vi "Chain3_bak.vi"(7 "Name (\"\" to Use UUID)":string="CSM-Module") -> ()   [LabVIEW 2017, in "CSM-Testcase.lvlib"]
doc: "Creates a template for a CSM module without a user interface.\n\n> [!NOTE] CSM Name Rules\n> - The CSM module name must be unique to avoid entering the \"Critical Error\" state.\n> - If the input is \"\", a UUID will be used as the module name. This module will operate in independent mode and will not be listed in the module list.\n> - If the input ends with '#', the module will run in work mode. Modules with the same name will share the same message queue. External messages will be handled by the idle module.\n\n> [!NOTE] CSM Initialization State\n> - The default value is \"Macro: Initialize\", consistent with the JKISM state machine.\n> - This state is typically not modified and is provided to facilitate external programmatic changes to the initialization state.\n\n\n-- <b>Controls</b> --\n- <b>Name (\"\" to Use UUID)</b>: CSM Module Name\n- <b>Init State(\"Macro: Initialize\")</b>: Initialization State, default is \"Macro: Initialize\""
uses:
  CSM-Testcase.lvlib
  250f9197-eaab-42aa-85f4-d19595f3ef40.vi
  b1f9a1d7-2f6f-40c5-bed8-42b286b8eb3f.vi
  e695532a-dccc-48b0-b567-f6fcd461bdfb.vi
  src/user.lib/_NEVSTOP/Communicable State Machine(CSM)/AdvanceAPI/CSM - Revert Arguments-Safe String.vi
  src/user.lib/_NEVSTOP/Communicable State Machine(CSM)/AdvanceAPI/CSM - Make String Arguments Safe.vi
  src/user.lib/_NEVSTOP/Communicable State Machine(CSM)/AdvanceAPI/CSM - Break Down Multiple States String.vi
  src/user.lib/_NEVSTOP/Communicable State Machine(CSM)/AdvanceAPI/CSM - Keywords.vi
  src/user.lib/_NEVSTOP/Communicable State Machine(CSM)/_Shared/Trim Single-line Text.vi
  Global-TestcaseCSM.vi
  src/user.lib/_NEVSTOP/Communicable State Machine(CSM)/_Polymophic/Build No-Reply Asynchronous Message with Arguments.vi
  src/user.lib/_NEVSTOP/Communicable State Machine(CSM)/_Polymophic/Build Asynchronous Message with Arguments.vi
  src/user.lib/_NEVSTOP/Communicable State Machine(CSM)/_Polymophic/Build Register Status Message.vi
  src/user.lib/_NEVSTOP/Communicable State Machine(CSM)/Communicable State Machine.lvlib
panel:
  out "Error Occurred":errorcluster
  out "State History":string
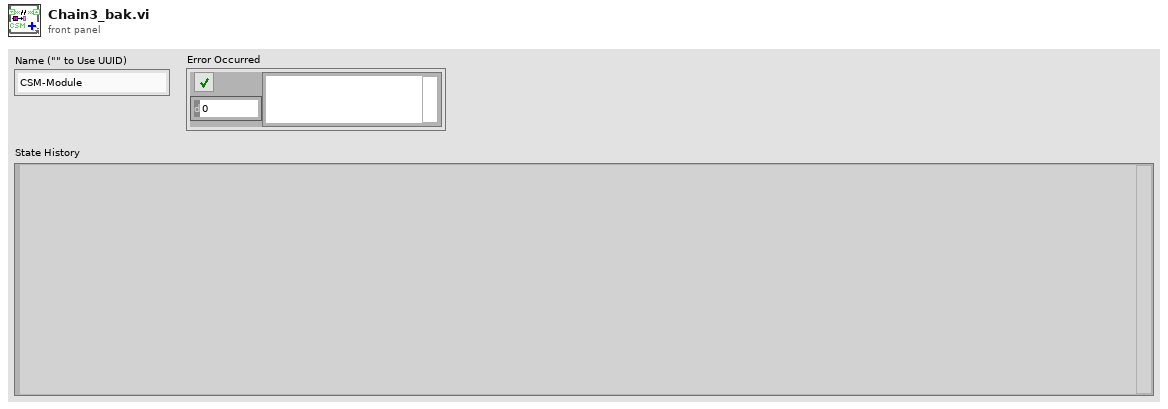
[diagram p1: front panel]
types:
  T1 = cluster{"Arguments":string, "Response":string, "error":errorcluster}
  T2 = enum32{"Invalid", "Standard", "Closed", "Hidden", "Minimized", "Maximized"}
  T3 = enum32{"invalid app kind", "Development System", "Run Time System", "Student Edition", "Embedded LabVIEW", "Evaluation", "Custom"}
  T4 = typedef "Communicable State Machine.lvlib/_CSM_Response Source Message.ctl" = cluster{"‘State":string, "’Arguments":string, "’Error":errorcluster}
  T5 = cluster{"Current VI Reference":refnum<vi>, "Close Panel on Exit?":bool}
  T6 = cluster{"Core":cluster{"Current VI Reference":refnum<vi>, "Close Panel on Exit?":bool}, "Your Boolean data":bool, "Your string data":string}
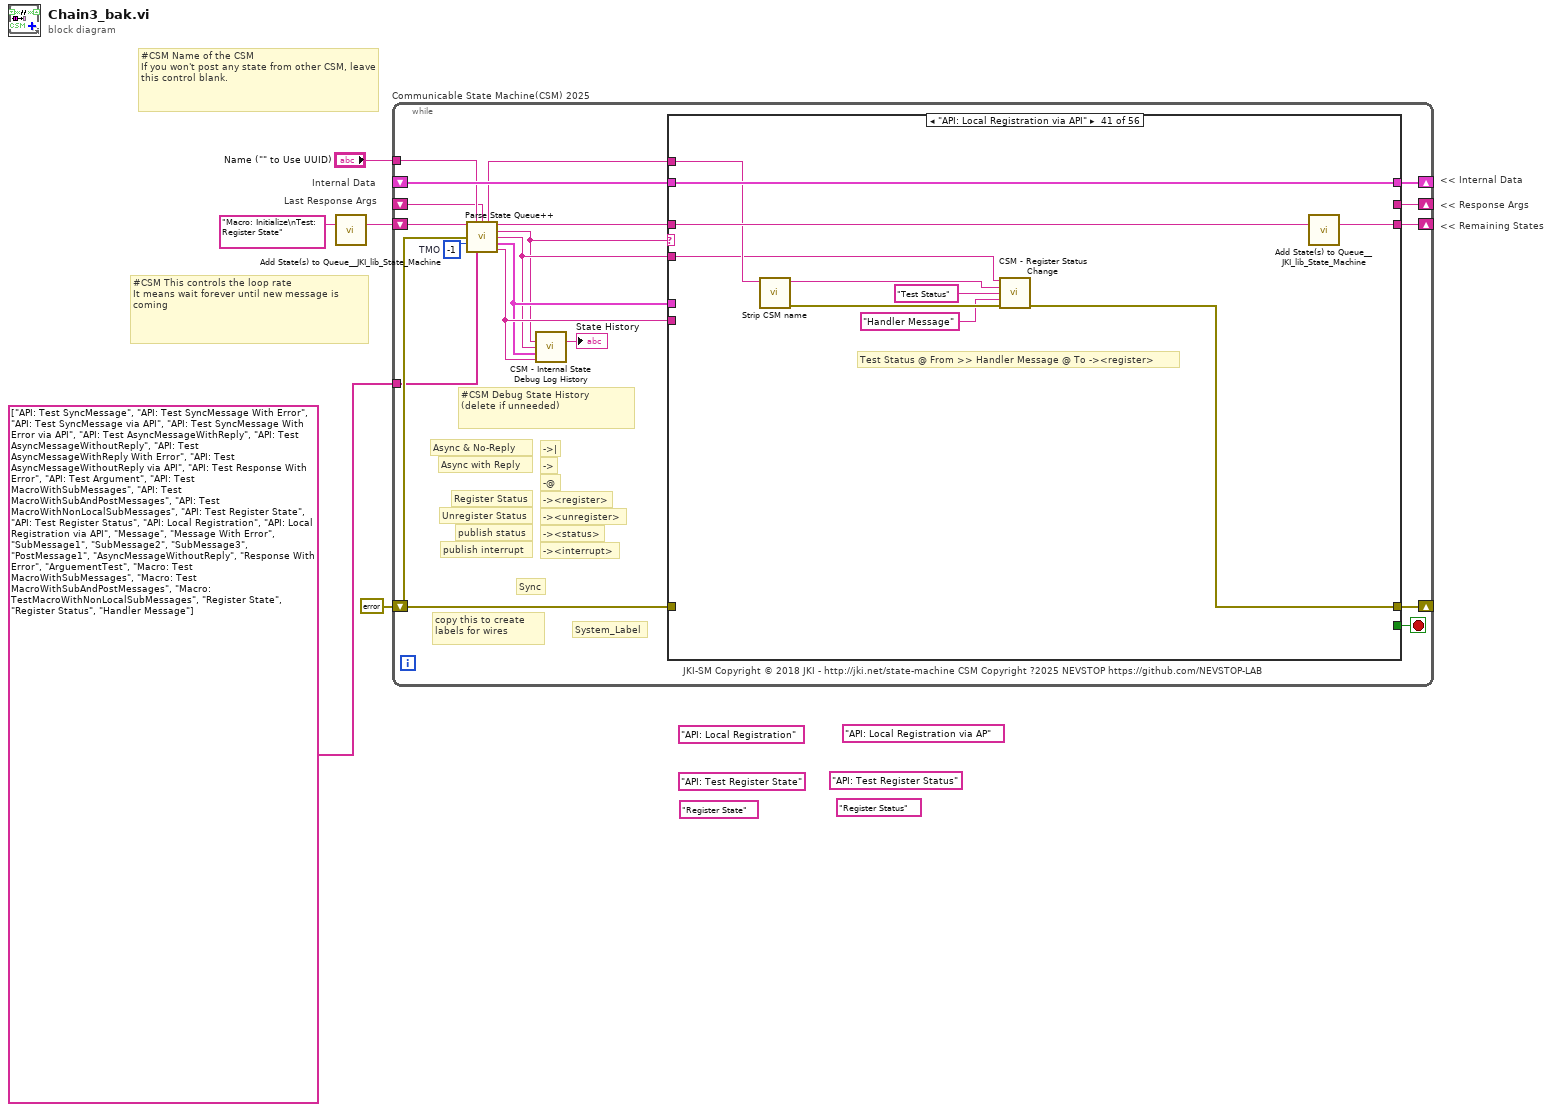
[diagram p0: block diagram]
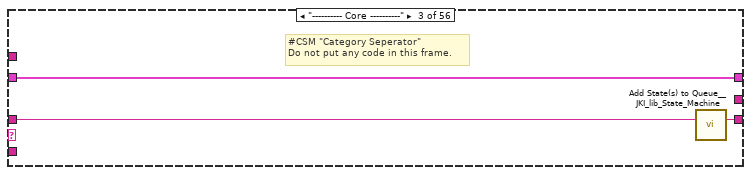
[diagram p4: hidden frame]
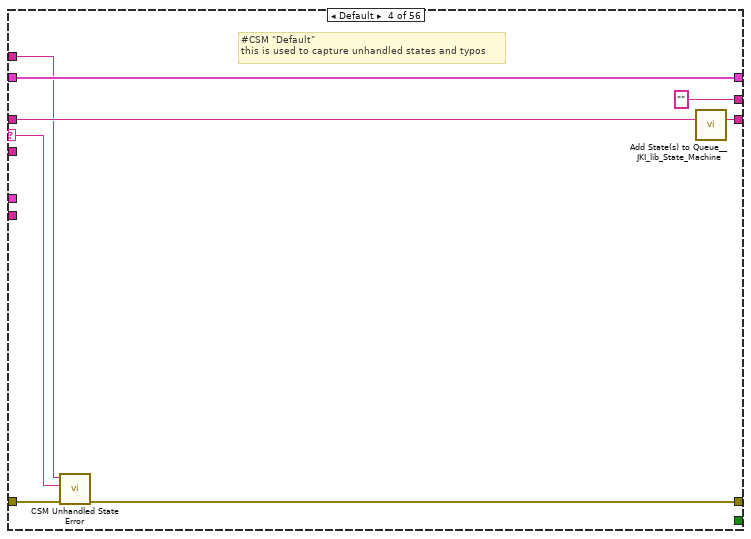
[diagram p5: hidden frame]
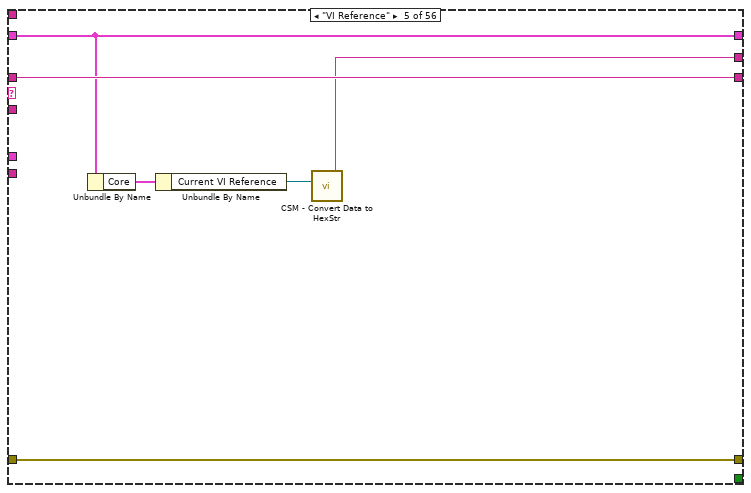
[diagram p6: hidden frame]
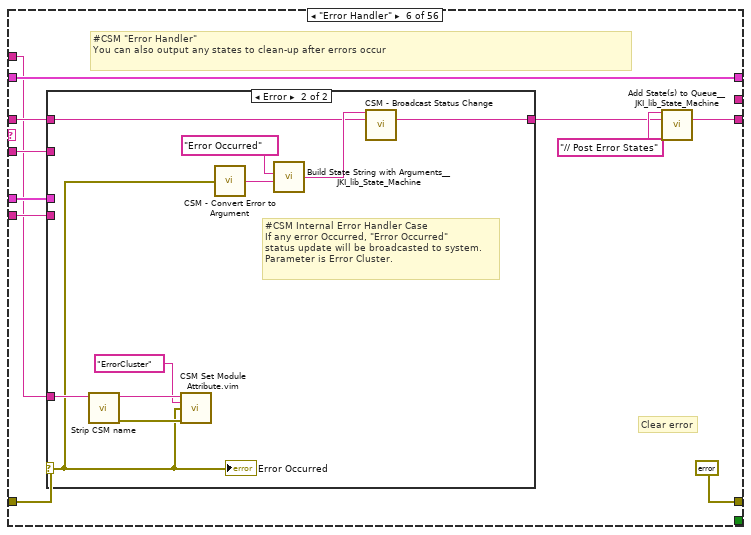
[diagram p7: hidden frame]
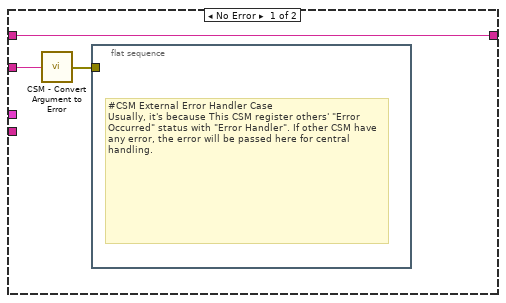
[diagram p8: hidden frame]
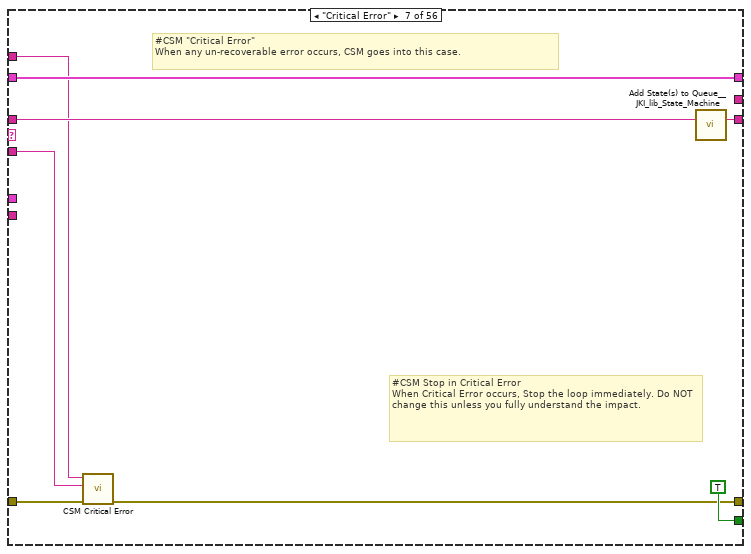
[diagram p9: hidden frame]
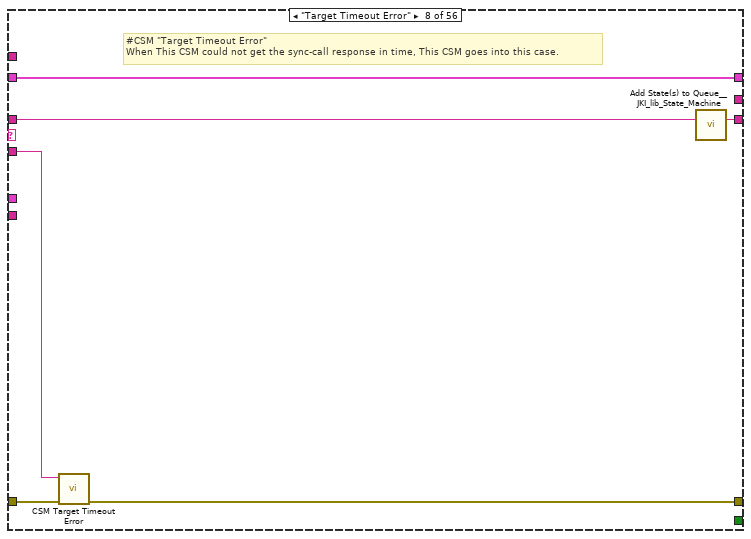
[diagram p10: hidden frame]
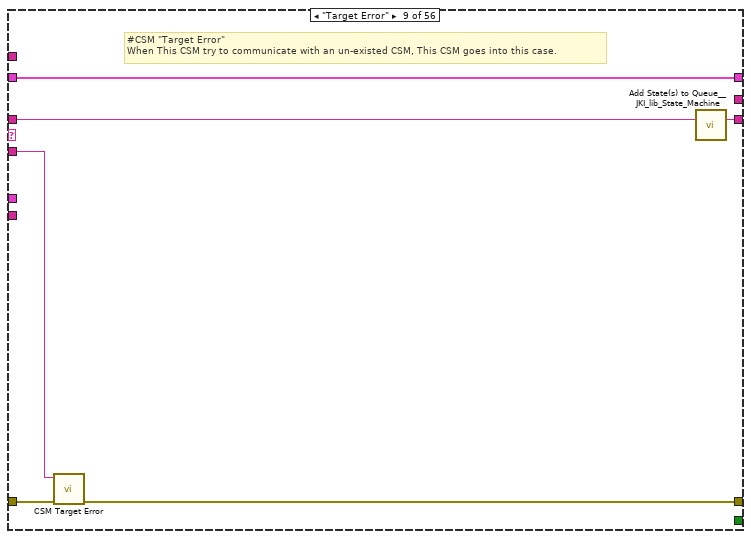
[diagram p11: hidden frame]
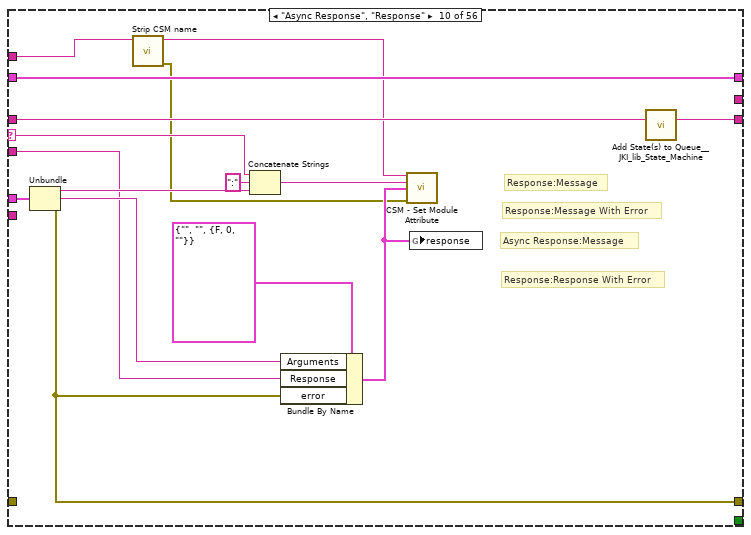
[diagram p12: hidden frame]
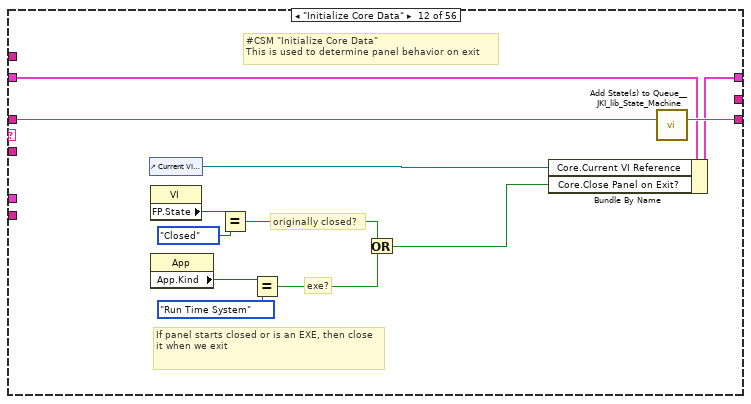
[diagram p14: hidden frame]
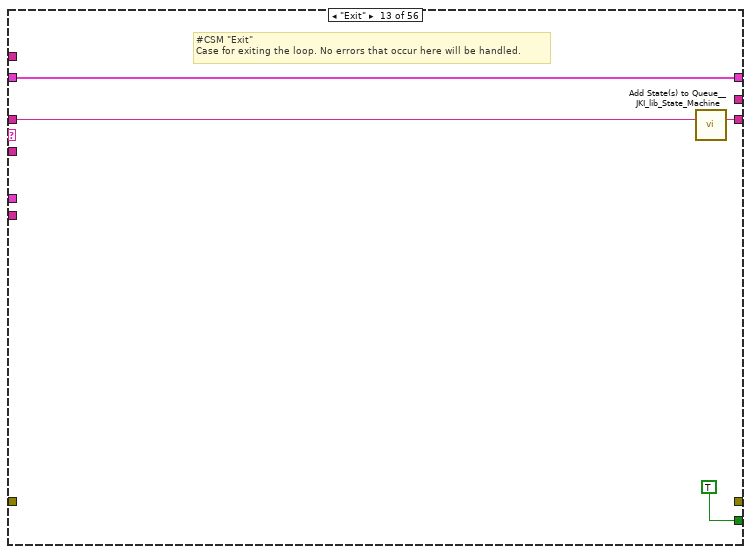
[diagram p15: hidden frame]
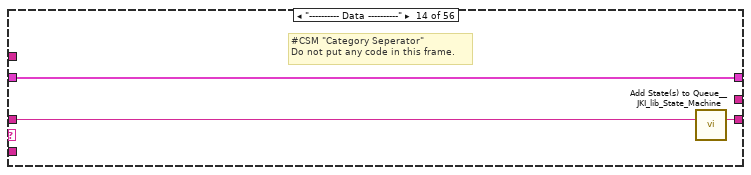
[diagram p16: hidden frame]
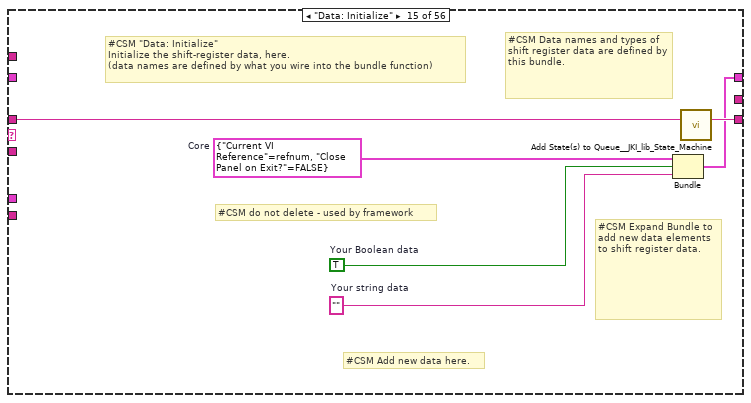
[diagram p17: hidden frame]
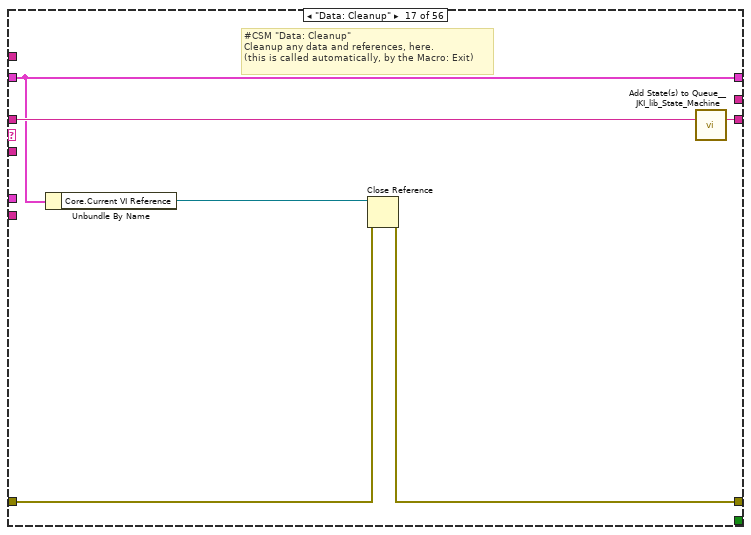
[diagram p19: hidden frame]
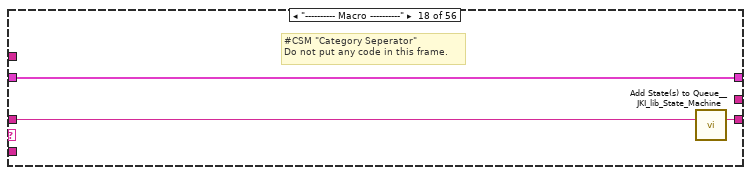
[diagram p20: hidden frame]
diagram:
  (unwired) "API: Local Registration via AP"
  (unwired) "API: Local Registration"
  (unwired) "API: Test Register Status"
  (unwired) "API: Test Register State"
  (unwired) "Register State"
  (unwired) "Register Status"
  # "Last Response Args"
  # "Internal Data"
  # "#CSM Name of the CSM\nIf you won't post any state from other CSM, leave this control blank."
  # "#CSM This controls the loop rate\nIt means wait forever until new message is coming"
  # "<< Internal Data"
  # "<< Response Args"
  # "<< Remaining States"
  n1 = call <vilib>:"Add State(s) to Queue__JKI_lib_State_Machine.vi"("State(s) in (\"\")"="Macro: Initialize\nTest: Register State" ("Init State(\"Macro: Initialize\")")) -> ("States Out"=w5:string)  [unwired: 14 in]
  n2 = while "Communicable State Machine(CSM) 2025" {
    shift-right: [w19] -> _
    shift-left: _ -> [w18]
    shift-right: [w22] -> _
    shift-left: errorcluster {"status"=FALSE, "code"=0, "source"=""} ("error out") -> [w8]
    shift-right: [w21] -> _
    shift-left: w5 -> [w23]
    tunnel: "Name (\"\" to Use UUID)" -> [w15]
    shift-right: [w16] -> _
    shift-left: _ -> [w10]
    tunnel: string[] ["API: Test SyncMessage", "API: Test SyncMessage With Error", "API: Test SyncMessage via API", "API: Test SyncMessage With Error via API", "API: Test AsyncMessageWithReply", "API: Test AsyncMessageWithoutReply", "API: Test AsyncMessageWithReply With Error", "API: Test AsyncMessageWithoutReply via API", "API: Test Response With Error", "API: Test Argument", "API: Test MacroWithSubMessages", "API: Test MacroWithSubAndPostMessages", "API: Test MacroWithNonLocalSubMessages", "API: Test Register State", "API: Test Register Status", "API: Local Registration", "API: Local Registration via API", "Message", "Message With Error", "SubMessage1", "SubMessage2", "SubMessage3", "PostMessage1", "AsyncMessageWithoutReply", "Response With Error", "ArguementTest", "Macro: Test MacroWithSubMessages", "Macro: Test MacroWithSubAndPostMessages", "Macro: TestMacroWithNonLocalSubMessages", "Register State", "Register Status", "Handler Message"] ("Allowed Messages (Empty for All)") -> [w6]
    stop <- w20 stop-if-true
    w17 = -1  # TMO
    # "#CSM Debug State History\n(delete if unneeded)"
    # "-><interrupt>"
    # "-><status>"
    # "-><unregister>"
    # "-><register>"
    # "-@"
    # "->"
    # "->|"
    # "publish interrupt"
    # "publish status"
    # "Unregister Status"
    # "Register Status"
    # "Sync"
    # "Async with Reply"
    # "Async & No-Reply"
    # "JKI-SM Copyright © 2018 JKI - http://jki.net/state-machine CSM Copyright ?2025 NEVSTOP https://github.com/NEVSTOP-LAB"
    # "copy this to create labels for wires"
    # "System_Label"
    n3 = call "Parse State Queue++.vi"("State Queue"=w23, "Name (\"\" to Use UUID)"=w15, "Response Arguments"=w10, "Previous Error"=w8, "Dequeue (1 ms)"=w17, "Allowed Messages (Empty for All)"=w6) -> ("Name Used"=w9:string, "Remaining States"=w24:string, "Current State"=w11:string, "Arguments"=w12:string, ">> Response Source Message >>"=w13:T4, ">> Source CSM >>"=w14:string)  [unwired: 4 in]
    n4 = call "CSM - Internal State Debug Log History.vi"("State"=w11, "Arguments (\"\")"=w12, ">> Response Source Message >>"=w13, "Source (\"\")"=w14) -> ("Debug Log"=→"State History":string)  [unwired: 11 in]
    n5 = case shown="\"API: Local Registration via API\"" w11 {
      selector: w11 -> [_ _ _ w35 _ _ _ _ _ w101 _ _ _ _ _ _ _ _ _ _ _ _ _ _ _ _ _ _ _ _ _ _ _ _ _ _ _ _ _ _ _ _ _ _ _ _ _ _ _ w487 _ _ _ w512 w525 w531]
      tunnel: w24 -> [w25 w28 w31 w39 w44 w50 w77 w83 w89 w105 w107 w119 w123 w126 w132 w134 w140 w143 w147 w153 w167 w187 w216 w220 w224 w236 w264 w296 w312 w324 w336 w350 w373 w384 w397 w404 w411 w418 w425 w437 w447 w451 w456 w459 w465 w470 w473 w477 w481 w491 w495 w503 w509 w517 w527 w537]
      tunnel: w12 -> [_ _ _ _ _ w49 w73 w80 w86 w95 _ _ _ _ _ _ _ _ _ _ w154 w174 w199 _ w227 w239 w267 w299 w315 w327 w339 w353 w369 w387 w394 w401 w408 w415 w422 w429 w438 w449 _ _ w461 w466 w472 w476 w480 w486 w494 w501 w507 w514 w526 w530]
      tunnel: w18 -> [w26 w27 w29 w37 w43 w55 w75 w81 w87 w103 w106 w113 w121 w124 _ w133 w135 w141 w145 w151 w169 w189 w218 w219 w228 w240 w268 w300 w316 w328 w340 w354 w376 w388 w399 w406 w413 w420 w427 w435 w445 w450 w454 w457 w463 w471 w474 w478 w482 w492 w496 w502 w508 w518 w528 w538]
      tunnel: [_ _ _ w32 w45 errorcluster {"status"=FALSE, "code"=0, "source"=""} ("error out") w70 w78 w84 w94 _ _ _ _ _ _ w136 _ _ _ _ _ _ _ w221 w233 w261 w293 w309 w321 w333 w346 w370 w381 w398 w405 w412 w419 w426 w431 w442 _ _ _ _ _ w475 w479 w483 w485 w497 w498 w504 w511 w521 w533] -> w22
      tunnel: w8 -> [_ _ _ w33 w45 w53 w71 w79 w85 _ _ _ _ _ _ _ w137 _ _ _ _ _ _ _ _ _ _ _ _ _ _ _ _ _ w398 w405 w412 w419 w426 _ _ _ _ _ _ _ w475 w479 w483 w493 w497 w499 w505 w519 w529 w539]
      tunnel: [w25 w28 w30 w38 w44 w51 w76 w82 w88 w104 w107 w118 w122 w125 w131 w134 w139 w142 w146 w152 w168 w188 w217 w220 w225 w237 w265 w297 w313 w325 w337 w351 w374 w385 w396 w403 w410 w417 w424 w436 w446 w451 w455 w458 w464 w467 w473 w477 w481 w491 w495 w503 w509 w517 w527 w537] -> w21
      tunnel: [_ _ _ _ _ _ TRUE _ _ _ _ _ TRUE _ _ _ _ _ _ _ _ _ _ _ _ _ _ _ _ _ _ _ _ _ _ _ _ _ _ _ _ _ _ _ _ _ _ _ _ _ _ _ _ _ _ _] -> w20
      tunnel: [w26 w27 w29 w37 w43 w55 w75 w81 w87 w103 w106 w117 w121 w124 w130 w133 w135 w141 w145 w151 w169 w189 w218 w219 w228 w240 w268 w300 w316 w328 w340 w354 w376 w388 w399 w406 w413 w420 w427 w435 w445 w450 w454 w457 w463 w471 w474 w478 w482 w492 w496 w502 w508 w518 w528 w538] -> w19
      tunnel: w14 -> [_ _ _ _ _ w48 _ _ _ _ _ _ _ _ _ _ _ _ _ _ _ _ _ _ _ _ _ _ _ _ _ _ _ _ _ _ _ _ _ _ _ _ _ _ _ _ _ _ _ _ _ _ _ _ _ _]
      tunnel: w13 -> [_ _ _ _ _ w47 _ _ _ w102 _ _ _ _ _ _ _ _ _ _ _ _ _ _ _ _ _ _ _ _ _ _ _ _ _ _ _ _ _ _ _ _ _ _ _ _ _ _ _ _ _ _ _ _ _ _]
      tunnel: [_ _ _ "" w40 _ _ _ _ _ _ _ _ _ _ _ _ _ _ _ _ _ _ _ _ _ _ _ _ _ _ _ _ _ _ _ _ _ _ _ _ w448 _ _ _ _ w472 w476 w480 w486 w494 w501 w507 _ w526 w530] -> w16
      tunnel: w9 -> [_ _ _ w34 _ w46 w72 _ _ w92 _ _ _ _ _ _ _ _ _ _ _ _ _ _ _ _ w252 w284 _ _ _ w347 _ _ _ _ _ _ _ w433 w444 _ _ _ _ _ _ _ _ w490 _ _ _ w516 w524 w536]
      frame "", "Idle" {
        # "#CSM \"Idle/Event Handler\"\nexecutes when the state queue is empty"
      }
      frame "CSM Documentation" {
        # "#CSM State Syntax\n\n// Comment line, all text to the right of “//” will be ignored\n// Local Message Example\nDoSth: DoA >> Arguments\n\n// Sync Call Example\nAPI: xxxx >> Arguments -@ TargetModule\n\n// Async Call Example\nAPI: xxxx >> Arguments -> TargetModule\n\n// Async Call without Reply Example\nAPI: xxxx >> Arguments ->| TargetModule\n\n// Broadcast normal status:\nStatus >> StatusArguments  -><status>\n\n// Broadcast Interrupt status:\nInterrupt >> StatusArguments  -><interrupt>\n\n// Register Source Module's status to Handler Module\nStatus@Source Module >> Handler Module@Handler Module -><register>\n\n// Unegister Source Module's status\nStatus@Source Module >> Handler Module -><unregister>"
        # "#CSM README FIRST\n\nCommunicable State Machine(CSM) is a LabVIEW application framework that builds upon JKI State Machine(JKISM). It follows the pattern of JKISM and extends the keywords to describe message communication between modules, including concepts such as Sync-Message, Async-Message, Subscription/Unsubscription of status - essential elements for creating reusable code modules. For more information, please visit the CSM wiki: https://nevstop-lab.github.io/CSM-Wiki/\n\nFor instructions on JKI State Machine, visit: \n    http://jki.net/state-machine/\nFor information about CSM, visit: \n    https://github.com/NEVSTOP-LAB"
        # "#CSM \"Documentation\"\nCase for holding CSM Documenation"
      }
      frame "---------- Core ----------" {
        # "#CSM \"Category Seperator\"\nDo not put any code in this frame."
        n6 = call <vilib>:"Add State(s) to Queue__JKI_lib_State_Machine.vi"("State(s) in (\"\")"=w31) -> ("States Out"=w30:string)  [unwired: 14 in]
      }
      frame Default {
        # "#CSM \"Default\"\nthis is used to capture unhandled states and typos"
        n7 = call "CSM Unhandled State Error.vi"("error in (no error)"=w33, "Current State"=w35, "CSM Name"=w34) -> ("error out"=w32:errorcluster)  [unwired: 8 in]
        n8 = call <vilib>:"Add State(s) to Queue__JKI_lib_State_Machine.vi"("State(s) in (\"\")"=w39) -> ("States Out"=w38:string)  [unwired: 14 in]
      }
      frame "VI Reference" {
        n9 = Unbundle By Name(w43) -> ("Core"=w42:T5)
        n10 = Unbundle By Name(w42) -> ("Current VI Reference"=w41:refnum<vi>)
        n11 = call "CSM - Convert Data to HexStr.vi"("Variant"=w41) -> ("HEX String (0-9,A-F)"=w40:string)  [unwired: 8 in]
      }
      frame "Error Handler" {
        # "#CSM \"Error Handler\"\nYou can also output any states to clean-up after errors occur"
        # "Clear error"
        n12 = case shown="Error" w53 {
          selector: w53 -> [_ w61]
          tunnel: [w59 w66] -> w52
          tunnel: w50 -> [w59 w65]
          tunnel: w49 -> [w58 _]
          tunnel: w48 -> [_ _]
          tunnel: w47 -> [_ _]
          tunnel: w46 -> [_ w64]
          frame No Error {
            n13 = call "CSM - Convert Argument to Error.vi"("Argument"=w58) -> ("Error"=w57:errorcluster)  [unwired: 4 in]
            n14 = flat-sequence {
              tunnel: w57 -> [_]
              frame #0 {
                # "#CSM External Error Handler Case\nUsually, it's because This CSM register others' \"Error Occurred\" status with \"Error Handler\". If other CSM have any error, the error will be passed here for central handling."
              }
            }
          }
          frame Error {
            # "#CSM Internal Error Handler Case \nIf any error Occurred, \"Error Occurred\" \nstatus update will be broadcasted to system.\nParameter is Error Cluster."
            n15 = call "Strip CSM name.vi"("CSM name"=w64) -> ("error out"=w63:errorcluster, "CSM name core"=w62:string)  [unwired: 7 in, 2 out]
            n16 = call "CSM Set Module Attribute.vim"("CSM Name"=w62, "Attribute"="ErrorCluster", "Value"=w61, "Error In"=w63) -> ()  [unwired: 8 in, 4 out]
            n17 = call "CSM - Convert Error to Argument.vi"("Error"=w61) -> ("Argument"=w68:string)  [unwired: 4 in]
            n18 = call <vilib>:"Build State String with Arguments__JKI_lib_State_Machine.vi"("Arguments (\"\")"=w68, "State"="Error Occurred" ("Status with Arguments")) -> ("State with Arguments"=w67:string)  [unwired: 4 in]
            n19 = call "CSM - Broadcast Status Change.vi"("Status With Arguments"=w67, "State Queue"=w65) -> ("Remaining States"=w66:string)  [unwired: 13 in]
            "Error Occurred" <- w61
          }
        }
        n20 = call <vilib>:"Add State(s) to Queue__JKI_lib_State_Machine.vi"("State(s) in Front (\"\")"="// Post Error States", "State(s) in (\"\")"=w52) -> ("States Out"=w51:string)  [unwired: 13 in]
      }
      frame "Critical Error" {
        # "#CSM \"Critical Error\"\nWhen any un-recoverable error occurs, CSM goes into this case."
        # "#CSM Stop in Critical Error\nWhen Critical Error occurs, Stop the loop immediately. Do NOT change this unless you fully understand the impact."
        n21 = call "CSM Critical Error.vi"("error in (no error)"=w71, "Arugments (As Reason)"=w73, "CSM Name"=w72) -> ("error out"=w70:errorcluster)  [unwired: 8 in]
        n22 = call <vilib>:"Add State(s) to Queue__JKI_lib_State_Machine.vi"("State(s) in (\"\")"=w77) -> ("States Out"=w76:string)  [unwired: 14 in]
      }
      frame "Target Timeout Error" {
        # "#CSM \"Target Timeout Error\"\nWhen This CSM could not get the sync-call response in time, This CSM goes into this case."
        n23 = call "CSM Target Timeout Error.vi"("error in (no error)"=w79, "Arguments (As CSM Name)"=w80) -> ("error out"=w78:errorcluster)  [unwired: 9 in]
        n24 = call <vilib>:"Add State(s) to Queue__JKI_lib_State_Machine.vi"("State(s) in (\"\")"=w83) -> ("States Out"=w82:string)  [unwired: 14 in]
      }
      frame "Target Error" {
        # "#CSM \"Target Error\"\nWhen This CSM try to communicate with an un-existed CSM, This CSM goes into this case."
        n25 = call "CSM Target Error.vi"("error in (no error)"=w85, "Arguments (As CSM Name)"=w86) -> ("error out"=w84:errorcluster)  [unwired: 9 in]
        n26 = call <vilib>:"Add State(s) to Queue__JKI_lib_State_Machine.vi"("State(s) in (\"\")"=w89) -> ("States Out"=w88:string)  [unwired: 14 in]
      }
      frame "Async Response", "Response" {
        # "Response:Response With Error"
        # "Response:Message With Error"
        # "Async Response:Message"
        # "Response:Message"
        n27 = Unbundle(w102) -> ("‘State"=w100:string, "’Arguments"=w96:string, "’Error"=w94:errorcluster)
        n28 = call "Strip CSM name.vi"("CSM name"=w92) -> ("error out"=w90:errorcluster, "CSM name core"=w91:string)  [unwired: 7 in, 2 out]
        n29 = Concatenate Strings(w101, ":" ("string"), w100) -> (w98:string)
        n30 = Bundle By Name(cluster=T1 {"Arguments"="", "Response"="", "error"={"status"=FALSE, "code"=0, "source"=""}}, "Arguments"=w96, "Response"=w95, "error"=w94) -> (w93:T1)
        n31 = call "CSM - Set Module Attribute.vi"("CSM Name"=w91, "Attribute"=w98, "Value"=w93, "Error In"=w90) -> ()  [unwired: 8 in, 4 out]
        n32 = global write "Global-TestcaseCSM.vi" "response"(w93) -> ()
        n33 = call <vilib>:"Add State(s) to Queue__JKI_lib_State_Machine.vi"("State(s) in (\"\")"=w105) -> ("States Out"=w104:string)  [unwired: 14 in]
      }
      frame "Async Message Posted" {
        # "#CSM \"Async Message Posted\"\nAfter Async Message is posted (-> or ->| ), CSM goes to this state for post-action.\nYou can use Argument - State to tell which Async Message is called."
      }
      frame "Initialize Core Data" {
        # "#CSM \"Initialize Core Data\"\nThis is used to determine panel behavior on exit"
        # "originally closed?"
        # "exe?"
        # "If panel starts closed or is an EXE, then close it when we exit"
        n34 = control-ref of="Current VI Reference"() -> (w111:refnum<vi>)
        n35 = property class="VI"() -> ("FP.State"=w110:T2)  [unwired: 2 in, 2 out]
        n36 = property class="App"() -> ("App.Kind"=w116:T3)  [unwired: 2 in, 2 out]
        n37 = Equal?(x=w110, y=T2."Closed" ("Front Panel Window:State")) -> (x = y?=w108:bool)
        n38 = Equal?(x=w116, y=T3."Run Time System" ("Application:Kind")) -> (x = y?=w114:bool)
        n39 = Or(x=w108, y=w114) -> (x .or. y?=w112:bool)
        n40 = Bundle By Name(cluster=w113, "Core.Current VI Reference"=w111, "Core.Close Panel on Exit?"=w112) -> (w117:T6)
        n41 = call <vilib>:"Add State(s) to Queue__JKI_lib_State_Machine.vi"("State(s) in (\"\")"=w119) -> ("States Out"=w118:string)  [unwired: 14 in]
      }
      frame "Exit" {
        # "#CSM \"Exit\"\nCase for exiting the loop. No errors that occur here will be handled."
        n42 = call <vilib>:"Add State(s) to Queue__JKI_lib_State_Machine.vi"("State(s) in (\"\")"=w123) -> ("States Out"=w122:string)  [unwired: 14 in]
      }
      frame "---------- Data ----------" {
        # "#CSM \"Category Seperator\"\nDo not put any code in this frame."
        n43 = call <vilib>:"Add State(s) to Queue__JKI_lib_State_Machine.vi"("State(s) in (\"\")"=w126) -> ("States Out"=w125:string)  [unwired: 14 in]
      }
      frame "Data: Initialize" {
        w127 = T5 {"Current VI Reference"=refnum, "Close Panel on Exit?"=FALSE}  # Core
        w129 = TRUE  # Your Boolean data
        w128 = ""  # Your string data
        # "#CSM \"Data: Initialize\"\nInitialize the shift-register data, here.\n(data names are defined by what you wire into the bundle function)"
        # "#CSM do not delete - used by framework"
        # "#CSM Expand Bundle to add new data elements to shift register data."
        # "#CSM Add new data here."
        # "#CSM Data names and types of shift register data are defined by this bundle."
        n44 = Bundle("Core"=w127, "Your Boolean data"=w129, "Your string data"=w128) -> (w130:T6)  [unwired: 1 in]
        n45 = call <vilib>:"Add State(s) to Queue__JKI_lib_State_Machine.vi"("State(s) in (\"\")"=w132) -> ("States Out"=w131:string)  [unwired: 14 in]
      }
      frame "Data: Update Indicators" {
      }
      frame "Data: Cleanup" {
        # "#CSM \"Data: Cleanup\"\nCleanup any data and references, here.\n(this is called automatically, by the Macro: Exit)"
        n46 = Unbundle By Name(w135) -> ("Core.Current VI Reference"=w138:refnum<vi>)
        n47 = Close Reference(reference=w138, error in (no error)=w137) -> (error out=w136:errorcluster)
        n48 = call <vilib>:"Add State(s) to Queue__JKI_lib_State_Machine.vi"("State(s) in (\"\")"=w140) -> ("States Out"=w139:string)  [unwired: 14 in]
      }
      frame "---------- Macro ----------" {
        # "#CSM \"Category Seperator\"\nDo not put any code in this frame."
        n49 = call <vilib>:"Add State(s) to Queue__JKI_lib_State_Machine.vi"("State(s) in (\"\")"=w143) -> ("States Out"=w142:string)  [unwired: 14 in]
      }
      frame "Macro: Initialize" {
        # "#CSM \"Macro: Initialize\"\nInitialization Macro (This is called once, when the VI starts)"
        n50 = call <vilib>:"Add State(s) to Queue__JKI_lib_State_Machine.vi"("State(s) in Front (\"\")"="Data: Initialize\nInitialize Core Data\nData: Update Indicators", "State(s) in (\"\")"=w147) -> ("States Out"=w146:string)  [unwired: 13 in]
      }
      frame "Macro: Exit" {
        # "#CSM \"Macro: Exit\"\nExit Macro (This is called once, when the VI exits)"
        n51 = call <vilib>:"Add State(s) to Queue__JKI_lib_State_Machine.vi"("State(s) in Front (\"\")"="//Exit Sub-Modules ", "State(s) at Back (\"\")"="Data: Cleanup\nExit") -> ("States Out"=w149:string)  [unwired: 13 in]
        n52 = call <vilib>:"Add State(s) to Queue__JKI_lib_State_Machine.vi"("State(s) in Front (\"\")"=w149, "State(s) in (\"\")"=w153) -> ("States Out"=w152:string)  [unwired: 13 in]
      }
      frame "Macro: Test MacroWithSubMessages" {
        w155 = "SubMessage2" ("State With Arguments")
        w157 = "SubMessage1" ("State With Arguments")
        n53 = call "uuid.vi"() -> ("UUID"=w156:string)  [unwired: 11 in]
        n54 = call "uuid.vi"() -> ("UUID"=w158:string)  [unwired: 11 in]
        n55 = Concatenate Strings(w157, w158) -> (w159:string)
        n56 = Concatenate Strings(w155, w156) -> (w160:string)
        n57 = call <vilib>:"Build State String with Arguments__JKI_lib_State_Machine.vi"("Arguments (\"\")"=w154, "State"="SubMessage3" ("State With Arguments")) -> ("State with Arguments"=w162:string)  [unwired: 4 in]
        n58 = call <vilib>:"Build State String with Arguments__JKI_lib_State_Machine.vi"("Arguments (\"\")"=w159, "State"=w157) -> ("State with Arguments"=w164:string)  [unwired: 4 in]
        n59 = call <vilib>:"Build State String with Arguments__JKI_lib_State_Machine.vi"("Arguments (\"\")"=w160, "State"=w155) -> ("State with Arguments"=w163:string)  [unwired: 4 in]
        n60 = Build Array(w164, w163, w162) -> (w161:string[])
        n61 = call "CSM - Compact Multiple States.vi"("Multiple States"=w161) -> ("States"=w166:string)  [unwired: 9 in]
        n62 = call <vilib>:"Add State(s) to Queue__JKI_lib_State_Machine.vi"("State(s) in Front (\"\")"=w166, "State(s) in (\"\")"=w167) -> ("States Out"=w168:string)  [unwired: 13 in]
      }
      frame "Macro: Test MacroWithSubAndPostMessages" {
        w173 = "PostMessage1" ("State With Arguments")
        w175 = "SubMessage2" ("State With Arguments")
        w177 = "SubMessage1" ("State With Arguments")
        n63 = call "uuid.vi"() -> ("UUID"=w176:string)  [unwired: 11 in]
        n64 = call "uuid.vi"() -> ("UUID"=w172:string)  [unwired: 11 in]
        n65 = call "uuid.vi"() -> ("UUID"=w178:string)  [unwired: 11 in]
        n66 = Concatenate Strings(w173, w172) -> (w171:string)
        n67 = Concatenate Strings(w177, w178) -> (w179:string)
        n68 = Concatenate Strings(w175, w176) -> (w180:string)
        n69 = call <vilib>:"Build State String with Arguments__JKI_lib_State_Machine.vi"("Arguments (\"\")"=w174, "State"="SubMessage3" ("State With Arguments")) -> ("State with Arguments"=w182:string)  [unwired: 4 in]
        n70 = call <vilib>:"Build State String with Arguments__JKI_lib_State_Machine.vi"("Arguments (\"\")"=w171, "State"=w173) -> ("State with Arguments"=w170:string)  [unwired: 4 in]
        n71 = call <vilib>:"Build State String with Arguments__JKI_lib_State_Machine.vi"("Arguments (\"\")"=w179, "State"=w177) -> ("State with Arguments"=w184:string)  [unwired: 4 in]
        n72 = call <vilib>:"Build State String with Arguments__JKI_lib_State_Machine.vi"("Arguments (\"\")"=w180, "State"=w175) -> ("State with Arguments"=w183:string)  [unwired: 4 in]
        n73 = Build Array(w184, w183, w182) -> (w181:string[])
        n74 = call "CSM - Compact Multiple States.vi"("Multiple States"=w181) -> ("States"=w186:string)  [unwired: 9 in]
        n75 = call <vilib>:"Add State(s) to Queue__JKI_lib_State_Machine.vi"("State(s) in Front (\"\")"=w186, "State(s) in (\"\")"=w187, "State(s) at Back (\"\")"=w170) -> ("States Out"=w188:string)  [unwired: 12 in]
      }
      frame "Macro: TestMacroWithNonLocalSubMessages" {
        w203 = "PostMessage1" ("State With Arguments")
        w204 = "SubMessage2" ("State With Arguments")
        w206 = "SubMessage1" ("State With Arguments")
        n76 = Match Pattern(string=w199, regular expression="+") -> (before substring=w191:string, after substring=w190:string)  [unwired: 1 in, 2 out]
        n77 = call "uuid.vi"() -> ("UUID"=w202:string)  [unwired: 11 in]
        n78 = call "uuid.vi"() -> ("UUID"=w205:string)  [unwired: 11 in]
        n79 = call "uuid.vi"() -> ("UUID"=w207:string)  [unwired: 11 in]
        n80 = Concatenate Strings(w203, w202) -> (w201:string)
        n81 = Concatenate Strings(w206, w207) -> (w208:string)
        n82 = Concatenate Strings(w204, w205) -> (w209:string)
        n83 = call <vilib>:"Build State String with Arguments__JKI_lib_State_Machine.vi"("Arguments (\"\")"=w201, "State"=w203) -> ("State with Arguments"=w200:string)  [unwired: 4 in]
        n84 = call-poly "Build Message with Arguments++.vi"("State With Arguments"="SubMessage1", "Target Module (\"\")"=w190) -> ("CSM Message String"=w195:string)  [unwired: 13 in]
        n85 = call-poly "Build Message with Arguments++.vi"("State With Arguments"="SubMessage2", "Target Module (\"\")"=w190) -> ("CSM Message String"=w194:string)  [unwired: 13 in]
        n86 = call <vilib>:"Build State String with Arguments__JKI_lib_State_Machine.vi"("Arguments (\"\")"=w191, "State"="SubMessage3" ("State With Arguments")) -> ("State with Arguments"=w211:string)  [unwired: 4 in]
        n87 = call-poly "Build Message with Arguments++.vi"("State With Arguments"="Message", "Target Module (\"\")"=w190) -> ("CSM Message String"=w196:string)  [unwired: 13 in]
        n88 = call <vilib>:"Build State String with Arguments__JKI_lib_State_Machine.vi"("Arguments (\"\")"=w208, "State"=w206) -> ("State with Arguments"=w213:string)  [unwired: 4 in]
        n89 = call <vilib>:"Build State String with Arguments__JKI_lib_State_Machine.vi"("Arguments (\"\")"=w209, "State"=w204) -> ("State with Arguments"=w212:string)  [unwired: 4 in]
        n90 = Build Array(w213, w212, w211, w196, w195, w194) -> (w210:string[])
        n91 = call "CSM - Compact Multiple States.vi"("Multiple States"=w210) -> ("States"=w215:string)  [unwired: 9 in]
        n92 = call <vilib>:"Add State(s) to Queue__JKI_lib_State_Machine.vi"("State(s) in Front (\"\")"=w215, "State(s) in (\"\")"=w216, "State(s) at Back (\"\")"=w200) -> ("States Out"=w217:string)  [unwired: 12 in]
      }
      frame "---------- API ----------" {
        # "#CSM \"Category Seperator\"\nDo not put any code in this frame."
      }
      frame "API: Test SyncMessage" {
        n93 = call "CSM - Check If Module Exists.vi"("CSM Name"=w227) -> ("error out"=w221:errorcluster, "Exist?"=w222:bool, "CSM Name (Dup)"=w226:string)  [unwired: 8 in]
        n94 = case shown="True" w222 {
          tunnel: w226 -> [_ w230]
          tunnel: [_ w229] -> w223
          frame False {
          }
          frame True {
            n95 = call "uuid.vi"() -> ("UUID"=w231:string)  [unwired: 11 in]
            n96 = call "Build Synchronous Message with Arguments.vi"("State With Arguments"="Message", "Arguments (\"\")"=w231, "Target Module (\"\")"=w230) -> ("CSM Message String"=w229:string)  [unwired: 12 in]
          }
        }
        n97 = call <vilib>:"Add State(s) to Queue__JKI_lib_State_Machine.vi"("State(s) in Front (\"\")"=w223, "State(s) in (\"\")"=w224) -> ("States Out"=w225:string)  [unwired: 13 in]
      }
      frame "API: Test SyncMessage With Error" {
        n98 = call "CSM - Check If Module Exists.vi"("CSM Name"=w239) -> ("error out"=w233:errorcluster, "Exist?"=w234:bool, "CSM Name (Dup)"=w238:string)  [unwired: 8 in]
        n99 = case shown="True" w234 {
          tunnel: w238 -> [_ w242]
          tunnel: [_ w241] -> w235
          frame False {
          }
          frame True {
            n100 = call "uuid.vi"() -> ("UUID"=w243:string)  [unwired: 11 in]
            n101 = call "Build Synchronous Message with Arguments.vi"("State With Arguments"="Message With Error", "Arguments (\"\")"=w243, "Target Module (\"\")"=w242) -> ("CSM Message String"=w241:string)  [unwired: 12 in]
          }
        }
        n102 = call <vilib>:"Add State(s) to Queue__JKI_lib_State_Machine.vi"("State(s) in Front (\"\")"=w235, "State(s) in (\"\")"=w236) -> ("States Out"=w237:string)  [unwired: 13 in]
      }
      frame "API: Test SyncMessage via API" {
        n103 = call "CSM - Check If Module Exists.vi"("CSM Name"=w267) -> ("error out"=w262:errorcluster, "Exist?"=w263:bool, "CSM Name (Dup)"=w266:string)  [unwired: 8 in]
        n104 = case shown="True" w263 {
          tunnel: w266 -> [_ w276]
          tunnel: [_ w275] -> w250
          tunnel: w252 -> [_ w274]
          tunnel: [_ w273] -> w259
          tunnel: [_ w272] -> w248
          tunnel: [_ w271] -> w255
          tunnel: [_ w270] -> w258
          frame False {
          }
          frame True {
            w273 = "Message" ("State With Arguments")
            n105 = call "uuid.vi"() -> ("UUID"=w271:string)  [unwired: 11 in]
            n106 = call "CSM - Wait and Send Message for Reply.vi"("State"=w273, "Current Module (\"\" to Generate an ID)"=w274, "Arguments (\"\")"=w271, "Target Module"=w276) -> ("Response"=w270:string, ">> Source CSM >>"=w272:string, "error out"=w275:errorcluster)  [unwired: 9 in]
          }
        }
        n107 = call "Strip CSM name.vi"("CSM name"=w252) -> ("error out"=w249:errorcluster, "CSM name core"=w251:string)  [unwired: 7 in, 2 out]
        n108 = call "Strip CSM name.vi"("CSM name"=w248) -> ("error out"=w245:errorcluster, "CSM name core"=w247:string)  [unwired: 7 in, 2 out]
        n109 = Bundle By Name(cluster=T1 {"Arguments"="", "Response"="", "error"={"status"=FALSE, "code"=0, "source"=""}}, "Arguments"=w255, "Response"=w258, "error"=w250) -> (w253:T1)
        n110 = Concatenate Strings(w247, ":" ("string"), w259) -> (w257:string)
        n111 = Merge Errors(w249, w245) -> (w246:errorcluster)
        n112 = call "CSM - Set Module Attribute.vi"("CSM Name"=w251, "Attribute"=w257, "Value"=w253, "Error In"=w246) -> ("error out"=w256:errorcluster)  [unwired: 8 in, 3 out]
        n113 = disable-structure shown="Enabled" {
          disable-tunnel: w253 -> [w269 _]
          frame Enabled {
            n114 = global write "Global-TestcaseCSM.vi" "response"(w269) -> ()
          }
          frame Disabled {
          }
        }
        n115 = call <vilib>:"Add State(s) to Queue__JKI_lib_State_Machine.vi"("State(s) in (\"\")"=w264) -> ("States Out"=w265:string)  [unwired: 14 in]
        n116 = Merge Errors(w256, w250, w262) -> (w261:errorcluster)
      }
      frame "API: Test SyncMessage With Error via API" {
        n117 = call "CSM - Check If Module Exists.vi"("CSM Name"=w299) -> ("error out"=w294:errorcluster, "Exist?"=w295:bool, "CSM Name (Dup)"=w298:string)  [unwired: 8 in]
        n118 = case shown="True" w295 {
          tunnel: w298 -> [_ w308]
          tunnel: [_ w307] -> w281
          tunnel: w284 -> [_ w306]
          tunnel: [_ w305] -> w291
          tunnel: [_ w304] -> w280
          tunnel: [_ w303] -> w287
          tunnel: [_ w302] -> w290
          frame False {
          }
          frame True {
            w305 = "Message With Error" ("State With Arguments")
            n119 = call "uuid.vi"() -> ("UUID"=w303:string)  [unwired: 11 in]
            n120 = call "CSM - Wait and Send Message for Reply.vi"("State"=w305, "Current Module (\"\" to Generate an ID)"=w306, "Arguments (\"\")"=w303, "Target Module"=w308) -> ("Response"=w302:string, ">> Source CSM >>"=w304:string, "error out"=w307:errorcluster)  [unwired: 9 in]
          }
        }
        n121 = call "Strip CSM name.vi"("CSM name"=w280) -> ("error out"=w277:errorcluster, "CSM name core"=w279:string)  [unwired: 7 in, 2 out]
        n122 = Bundle By Name(cluster=T1 {"Arguments"="", "Response"="", "error"={"status"=FALSE, "code"=0, "source"=""}}, "Arguments"=w287, "Response"=w290, "error"=w281) -> (w286:T1)
        n123 = call "Strip CSM name.vi"("CSM name"=w284) -> ("error out"=w282:errorcluster, "CSM name core"=w283:string)  [unwired: 7 in, 2 out]
        n124 = Concatenate Strings(w279, ":" ("string"), w291) -> (w289:string)
        n125 = Merge Errors(w282, w277) -> (w278:errorcluster)
        n126 = disable-structure shown="Enabled" {
          disable-tunnel: w286 -> [w301 _]
          frame Enabled {
            n127 = global write "Global-TestcaseCSM.vi" "response"(w301) -> ()
          }
          frame Disabled {
          }
        }
        n128 = call "CSM - Set Module Attribute.vi"("CSM Name"=w283, "Attribute"=w289, "Value"=w286, "Error In"=w278) -> ("error out"=w288:errorcluster)  [unwired: 8 in, 3 out]
        n129 = call <vilib>:"Add State(s) to Queue__JKI_lib_State_Machine.vi"("State(s) in (\"\")"=w296) -> ("States Out"=w297:string)  [unwired: 14 in]
        n130 = Merge Errors(w288, w281, w294) -> (w293:errorcluster)
      }
      frame "API: Test AsyncMessageWithReply" {
        n131 = call "CSM - Check If Module Exists.vi"("CSM Name"=w315) -> ("error out"=w309:errorcluster, "Exist?"=w310:bool, "CSM Name (Dup)"=w314:string)  [unwired: 8 in]
        n132 = case shown="True" w310 {
          tunnel: w314 -> [_ w318]
          tunnel: [_ w317] -> w311
          frame False {
          }
          frame True {
            n133 = call "uuid.vi"() -> ("UUID"=w319:string)  [unwired: 11 in]
            n134 = call-poly "Build Message with Arguments++.vi"("State With Arguments"="Message", "Arguments (\"\")"=w319, "Target Module (\"\")"=w318) -> ("CSM Message String"=w317:string)  [unwired: 12 in]
          }
        }
        n135 = call <vilib>:"Add State(s) to Queue__JKI_lib_State_Machine.vi"("State(s) in Front (\"\")"=w311, "State(s) in (\"\")"=w312) -> ("States Out"=w313:string)  [unwired: 13 in]
      }
      frame "API: Test AsyncMessageWithReply With Error" {
        n136 = call "CSM - Check If Module Exists.vi"("CSM Name"=w327) -> ("error out"=w321:errorcluster, "Exist?"=w322:bool, "CSM Name (Dup)"=w326:string)  [unwired: 8 in]
        n137 = case shown="True" w322 {
          tunnel: w326 -> [_ w331]
          tunnel: [_ w329] -> w323
          frame False {
          }
          frame True {
            n138 = call "uuid.vi"() -> ("UUID"=w330:string)  [unwired: 11 in]
            n139 = call-poly "Build Message with Arguments++.vi"("State With Arguments"="Message With Error", "Arguments (\"\")"=w330, "Target Module (\"\")"=w331) -> ("CSM Message String"=w329:string)  [unwired: 12 in]
          }
        }
        n140 = call <vilib>:"Add State(s) to Queue__JKI_lib_State_Machine.vi"("State(s) in Front (\"\")"=w323, "State(s) in (\"\")"=w324) -> ("States Out"=w325:string)  [unwired: 13 in]
      }
      frame "API: Test AsyncMessageWithoutReply" {
        n141 = call "CSM - Check If Module Exists.vi"("CSM Name"=w339) -> ("error out"=w333:errorcluster, "Exist?"=w334:bool, "CSM Name (Dup)"=w338:string)  [unwired: 8 in]
        n142 = case shown="True" w334 {
          tunnel: w338 -> [_ w344]
          tunnel: [_ w342] -> w335
          frame False {
          }
          frame True {
            n143 = call-poly "Build Message with Arguments++.vi"("State With Arguments"="AsyncMessageWithoutReply", "Arguments (\"\")"="123456789" ("Arguments (\"\")"), "Target Module (\"\")"=w344) -> ("CSM Message String"=w342:string)  [unwired: 12 in]
          }
        }
        n144 = call <vilib>:"Add State(s) to Queue__JKI_lib_State_Machine.vi"("State(s) in Front (\"\")"=w335, "State(s) in (\"\")"=w336) -> ("States Out"=w337:string)  [unwired: 13 in]
      }
      frame "API: Test AsyncMessageWithoutReply via API" {
        n145 = call "CSM - Check If Module Exists.vi"("CSM Name"=w353) -> ("error out"=w348:errorcluster, "Exist?"=w349:bool, "CSM Name (Dup)"=w352:string)  [unwired: 8 in]
        n146 = case shown="True" w349 {
          tunnel: w352 -> [_ w356]
          tunnel: w347 -> [_ w359]
          tunnel: [_ w355] -> w345
          frame False {
          }
          frame True {
            n147 = call "CSM - Wait and Post Message.vi"("State"="AsyncMessageWithoutReply" ("State With Arguments"), "Current Module (\"\" to Generate an ID)"=w359, "Arguments (\"\")"="123456789" ("Arguments (\"\")"), "Target Module"=w356) -> ("error out"=w355:errorcluster)  [unwired: 11 in]
          }
        }
        n148 = call <vilib>:"Add State(s) to Queue__JKI_lib_State_Machine.vi"("State(s) in (\"\")"=w350) -> ("States Out"=w351:string)  [unwired: 14 in]
        n149 = Merge Errors(w345, w348) -> (w346:errorcluster)
      }
      frame "API: Test Argument" {
        n150 = call "uuid.vi"() -> ("UUID"=w365:string)  [unwired: 11 in]
        n151 = call "CSM - Convert HexStr to Data.vi"("HEX String"=w369) -> ("Variant"=w367:variant, "error out"=w368:errorcluster)  [unwired: 7 in]
        n152 = Bundle("", "UUID"=w365) -> (w363:cluster{string, "UUID":string})  [unwired: 1 in]
        n153 = Variant To Data(error in=w368, type=w363, Variant=w367) -> (data=w362:cluster{string, "UUID":string}, error out=w366:errorcluster)
        n154 = Unbundle(w362) -> (w361:string, "UUID"=w360:string)
        n155 = call "CSM - Check If Module Exists.vi"("Error In"=w366, "CSM Name"=w361) -> ("error out"=w370:errorcluster, "Exist?"=w371:bool, "CSM Name (Dup)"=w375:string)  [unwired: 7 in]
        n156 = case shown="True" w371 {
          tunnel: w375 -> [_ w379]
          tunnel: [_ w378] -> w372
          tunnel: w360 -> [_ w377]
          frame False {
          }
          frame True {
            n157 = call "Build Synchronous Message with Arguments.vi"("State With Arguments"="ArgumentTest", "Arguments (\"\")"=w377, "Target Module (\"\")"=w379) -> ("CSM Message String"=w378:string)  [unwired: 12 in]
          }
        }
        n158 = call <vilib>:"Add State(s) to Queue__JKI_lib_State_Machine.vi"("State(s) in Front (\"\")"=w372, "State(s) in (\"\")"=w373) -> ("States Out"=w374:string)  [unwired: 13 in]
      }
      frame "API: Test Response With Error" {
        n159 = call "CSM - Check If Module Exists.vi"("CSM Name"=w387) -> ("error out"=w381:errorcluster, "Exist?"=w382:bool, "CSM Name (Dup)"=w386:string)  [unwired: 8 in]
        n160 = case shown="True" w382 {
          tunnel: w386 -> [_ w390]
          tunnel: [_ w389] -> w383
          frame False {
          }
          frame True {
            n161 = call "uuid.vi"() -> ("UUID"=w391:string)  [unwired: 11 in]
            n162 = call "Build Synchronous Message with Arguments.vi"("State With Arguments"="Response With Error", "Arguments (\"\")"=w391, "Target Module (\"\")"=w390) -> ("CSM Message String"=w389:string)  [unwired: 12 in]
          }
        }
        n163 = call <vilib>:"Add State(s) to Queue__JKI_lib_State_Machine.vi"("State(s) in Front (\"\")"=w383, "State(s) in (\"\")"=w384) -> ("States Out"=w385:string)  [unwired: 13 in]
      }
      frame "API: Test MacroWithSubMessages" {
        n164 = call <vilib>:"Build State String with Arguments__JKI_lib_State_Machine.vi"("Arguments (\"\")"=w394, "State"="Macro: Test MacroWithSubMessages") -> ("State with Arguments"=w393:string)  [unwired: 4 in]
        n165 = call <vilib>:"Add State(s) to Queue__JKI_lib_State_Machine.vi"("State(s) in Front (\"\")"=w393, "State(s) in (\"\")"=w397) -> ("States Out"=w396:string)  [unwired: 13 in]
      }
      frame "API: Test MacroWithSubAndPostMessages" {
        n166 = call <vilib>:"Build State String with Arguments__JKI_lib_State_Machine.vi"("Arguments (\"\")"=w401, "State"="Macro: Test MacroWithSubAndPostMessages") -> ("State with Arguments"=w400:string)  [unwired: 4 in]
        n167 = call <vilib>:"Add State(s) to Queue__JKI_lib_State_Machine.vi"("State(s) in Front (\"\")"=w400, "State(s) in (\"\")"=w404) -> ("States Out"=w403:string)  [unwired: 13 in]
      }
      frame "API: Test MacroWithNonLocalSubMessages" {
        n168 = call <vilib>:"Build State String with Arguments__JKI_lib_State_Machine.vi"("Arguments (\"\")"=w408, "State"="Macro: TestMacroWithNonLocalSubMessages") -> ("State with Arguments"=w407:string)  [unwired: 4 in]
        n169 = call <vilib>:"Add State(s) to Queue__JKI_lib_State_Machine.vi"("State(s) in Front (\"\")"=w407, "State(s) in (\"\")"=w411) -> ("States Out"=w410:string)  [unwired: 13 in]
      }
      frame "API: Test Register State" {
        n170 = call <vilib>:"Build State String with Arguments__JKI_lib_State_Machine.vi"("Arguments (\"\")"=w415, "State"="Register State") -> ("State with Arguments"=w414:string)  [unwired: 4 in]
        n171 = call <vilib>:"Add State(s) to Queue__JKI_lib_State_Machine.vi"("State(s) in Front (\"\")"=w414, "State(s) in (\"\")"=w418) -> ("States Out"=w417:string)  [unwired: 13 in]
      }
      frame "API: Test Register Status" {
        n172 = call <vilib>:"Build State String with Arguments__JKI_lib_State_Machine.vi"("Arguments (\"\")"=w422, "State"="Register Status") -> ("State with Arguments"=w421:string)  [unwired: 4 in]
        n173 = call <vilib>:"Add State(s) to Queue__JKI_lib_State_Machine.vi"("State(s) in Front (\"\")"=w421, "State(s) in (\"\")"=w425) -> ("States Out"=w424:string)  [unwired: 13 in]
      }
      frame "API: Local Registration" {
        # "Test Status @ From >> Handler Message @ To -><register>"
        n174 = call "Strip CSM name.vi"("CSM name"=w433) -> ("error out"=w431:errorcluster, "CSM name core"=w428:string)  [unwired: 7 in, 2 out]
        n175 = call-poly "Build Message with Arguments++.vi"("Target CSM"=w429, "Source CSM (* as Default)"=w428, "Status"="Test Status", "API (If \"\", Same As \"Status\")"="Handler Message") -> ("CSM Message String"=w430:string)  [unwired: 11 in]
        n176 = call <vilib>:"Add State(s) to Queue__JKI_lib_State_Machine.vi"("State(s) in Front (\"\")"=w430, "State(s) in (\"\")"=w437) -> ("States Out"=w436:string)  [unwired: 13 in]
      }
      frame "API: Local Registration via API" {
        # "Test Status @ From >> Handler Message @ To -><register>"
        n177 = call "Strip CSM name.vi"("CSM name"=w444) -> ("error out"=w443:errorcluster, "CSM name core"=w439:string)  [unwired: 7 in, 2 out]
        n178 = call "CSM - Register Status Change.vi"("CSM Name"=w438, "Source CSM Name (* as Default)"=w439, "Status"="Test Status", "Response Message (If \"\", Same as Source Message)"="Handler Message", "Error In"=w443) -> ("error out"=w442:errorcluster)  [unwired: 9 in, 1 out]
        n179 = call <vilib>:"Add State(s) to Queue__JKI_lib_State_Machine.vi"("State(s) in (\"\")"=w447) -> ("States Out"=w446:string)  [unwired: 14 in]
      }
      frame "API: API2" {
        # "#CSM API Example\nCopy/Rename this case for your own API"
        # "unpack Hex String  to Variant\nif complex parameter is needed."
        n180 = call "CSM - Convert HexStr to Data.vi"("HEX String"=w449) -> ()  [unwired: 7 in, 2 out]
        n181 = disable-structure shown="Disabled" {
          disable-tunnel: [w452 "API2 Response"] -> w448
          frame Disabled {
            # "pack variant to hexstr \nif complex response is needed."
            # "complex Response"
            n182 = call "CSM - Convert Data to HexStr.vi"() -> ("HEX String (0-9,A-F)"=w452:string)  [unwired: 9 in]
          }
          frame Enabled {
          }
        }
      }
      frame "---------- Action ----------" {
        # "#CSM \"Category Seperator\"\nDo not put any code in this frame."
        n183 = call <vilib>:"Add State(s) to Queue__JKI_lib_State_Machine.vi"("State(s) in (\"\")"=w456) -> ("States Out"=w455:string)  [unwired: 14 in]
      }
      frame "Action: action1" {
        # "#CSM \"Internal State\"\nThis category is used for holding internal states"
        n184 = call <vilib>:"Add State(s) to Queue__JKI_lib_State_Machine.vi"("State(s) in (\"\")"=w459) -> ("States Out"=w458:string)  [unwired: 14 in]
      }
      frame "Register State" {
        n185 = call <vilib>:"Build State String with Arguments__JKI_lib_State_Machine.vi"("Arguments (\"\")"=w461, "State"="Register Status" ("State(s) in Front (\"\")")) -> ("State with Arguments"=w460:string)  [unwired: 4 in]
        n186 = call <vilib>:"Add State(s) to Queue__JKI_lib_State_Machine.vi"("State(s) in Front (\"\")"=w460, "State(s) in (\"\")"=w465) -> ("States Out"=w464:string)  [unwired: 13 in]
      }
      frame "Register Status" {
        n187 = call <vilib>:"Build State String with Arguments__JKI_lib_State_Machine.vi"("Arguments (\"\")"=w466, "State"="Test Status") -> ("State with Arguments"=w468:string)  [unwired: 4 in]
        n188 = call "CSM - Broadcast Status Change.vi"("Status With Arguments"=w468, "State Queue"=w470) -> ("Remaining States"=w467:string)  [unwired: 13 in]
      }
      frame "Message" {
      }
      frame "SubMessage1" {
      }
      frame "SubMessage2" {
      }
      frame "SubMessage3" {
        n189 = call "Strip CSM name.vi"("CSM name"=w490) -> ("error out"=w488:errorcluster, "CSM name core"=w489:string)  [unwired: 7 in, 2 out]
        n190 = call "CSM - Set Module Attribute.vi"("CSM Name"=w489, "Attribute"=w487, "Value"=w486, "Error In"=w488) -> ("error out"=w484:errorcluster)  [unwired: 8 in, 3 out]
        n191 = Merge Errors(w484, w493) -> (w485:errorcluster)
      }
      frame "PostMessage1" {
      }
      frame "Message With Error" {
        n192 = Merge Errors(errorcluster {"status"=TRUE, "code"=1234567898, "source"="Simulated Error\nwill be sent to Response case"} ("error out"), w499) -> (w498:errorcluster)
      }
      frame "Response With Error" {
        n193 = Merge Errors(errorcluster {"status"=TRUE, "code"=1234567898, "source"="Simulated Error"} ("error out"), w505) -> (w504:errorcluster)
      }
      frame "ArgumentTest" {
        n194 = call "Strip CSM name.vi"("CSM name"=w516) -> ("error out"=w513:errorcluster, "CSM name core"=w515:string)  [unwired: 7 in, 2 out]
        n195 = call "CSM Set Module Attribute.vim"("CSM Name"=w515, "Attribute"=w512, "Value"=w514, "Error In"=w513) -> ("error out"=w510:errorcluster)  [unwired: 8 in, 3 out]
        n196 = Merge Errors(w510, w519) -> (w511:errorcluster)
      }
      frame "AsyncMessageWithoutReply" {
        # "123456789 string constant"
        n197 = call "Strip CSM name.vi"("CSM name"=w524) -> ("error out"=w522:errorcluster, "CSM name core"=w523:string)  [unwired: 7 in, 2 out]
        n198 = call "CSM - Set Module Attribute.vi"("CSM Name"=w523, "Attribute"=w525, "Value"=w526, "Error In"=w522) -> ("error out"=w520:errorcluster)  [unwired: 8 in, 3 out]
        n199 = Merge Errors(w520, w529) -> (w521:errorcluster)
      }
      frame "Handler Message" {
        n200 = call "Strip CSM name.vi"("CSM name"=w536) -> ("error out"=w534:errorcluster, "CSM name core"=w535:string)  [unwired: 7 in, 2 out]
        n201 = call "CSM Set Module Attribute.vim"("CSM Name"=w535, "Attribute"=w531, "Value"=w530, "Error In"=w534) -> ("error out"=w532:errorcluster)  [unwired: 8 in, 3 out]
        n202 = Merge Errors(w532, w539) -> (w533:errorcluster)
      }
    }
  }
